vi "Configure Instrument.vi"(0 "Instrument Handle In":refnum<k21>, 5 "Instrument Configuration":T1, 11 "error in (no error)":errorcluster) -> (4 "Instrument Handle Out":refnum<k21>, 15 "error out":errorcluster)   [LabVIEW 2016, in "RFmxInstr.lvlib"]
uses:
  RFmxInstr.lvlib
  Typedefs/Instrument Configuration.ctl
  Common/Local Oscillator Sharing Mode.ctl
  <resource>/objmgr/RFmxInstr.rc
  Common/Common.lvlib
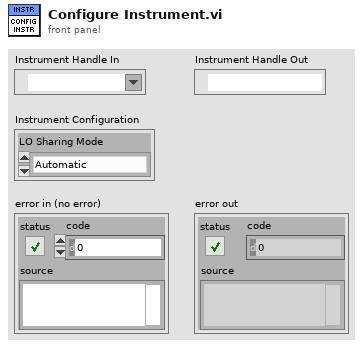
[diagram p1: front panel]
types:
  T1 = typedef "RFmxInstr.lvlib/Instrument Configuration.ctl" = cluster{"LO Sharing Mode":T2}
  T2 = typedef "Common.lvlib/Local Oscillator Sharing Mode.ctl" = enum16{"Automatic", "None"}
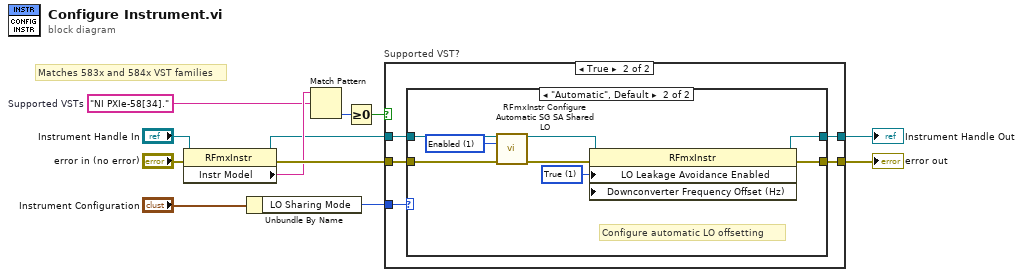
[diagram p0: block diagram]
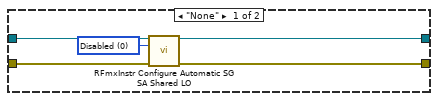
[diagram p3: hidden frame]
diagram:
  w9 = "NI PXIe-58[34]."  # Supported VSTs
  # "Matches 583x and 584x VST families"
  n1 = property class="RFmxInstr"(reference="Instrument Handle In", error in="error in (no error)") -> (reference out=w5:refnum<k21>, error out=w12:errorcluster, "Instr Model"=w10:string)
  n2 = Unbundle By Name("Instrument Configuration") -> ("LO Sharing Mode"=w1:T2)
  n3 = Match Pattern(string=w10, regular expression=w9) -> (offset past match=w8:i32)  [unwired: 1 in, 3 out]
  n4 = Greater Or Equal To 0?(x=w8) -> (x >= 0?=w3:bool)
  n5 = case "Supported VST?" shown="True" w3 {
    tunnel: [w14 w18] -> w7
    tunnel: w12 -> [w13 w15]
    tunnel: [w13 w19] -> w6
    tunnel: w5 -> [w14 w16]
    tunnel: w1 -> [_ w17]
    frame False {
      # "Do nothing; any configuration for LOs with standalone VSAs should be configured manually. Baseband instruments don't have LOs. Unsupported VSTs must be configured manually."
    }
    frame True {
      n6 = case shown="\"Automatic\", Default" w17 {
        tunnel: [w21 w32] -> w19
        tunnel: [w22 w25] -> w18
        tunnel: w16 -> [w24 w30]
        tunnel: w15 -> [w23 w29]
        frame "None" {
          w20 = 0 items=["Disabled", "Enabled"] ("Automatic SG SA Shared LO")
          n7 = call <vilib>:"RFmxInstr Configure Automatic SG SA Shared LO.vi"("Instrument Handle In"=w24, "Automatic SG SA Shared LO"=w20, "error in (no error)"=w23) -> ("Instrument Handle Out"=w22:refnum<k21>, "error out"=w21:errorcluster)  [unwired: 11 in]
        }
        frame "Automatic", Default {
          w26 = 1 items=["Disabled", "Enabled"] ("Automatic SG SA Shared LO")
          w31 = 1 items=["False", "True"] ("LO Leakage Avoidance Enabled")
          # "Configure automatic LO offsetting"
          n8 = call <vilib>:"RFmxInstr Configure Automatic SG SA Shared LO.vi"("Instrument Handle In"=w30, "Automatic SG SA Shared LO"=w26, "error in (no error)"=w29) -> ("Instrument Handle Out"=w27:refnum<k21>, "error out"=w28:errorcluster)  [unwired: 11 in]
          n9 = property class="RFmxInstr" props=["LO Leakage Avoidance Enabled", "Downconverter Frequency Offset (Hz)"](reference=w27, error in=w28, "LO Leakage Avoidance Enabled"=w31) -> (reference out=w25:refnum<k21>, error out=w32:errorcluster)  [unwired: 1 in]
        }
      }
    }
  }
  "error out" <- w6
  "Instrument Handle Out" <- w7
